vi "Validate IP Address.vi"(4 "Error In":errorcluster, 5 "IP Address":string) -> (0 "Error Out":errorcluster, 1 "IP Address Out":string)   [LabVIEW 2013]
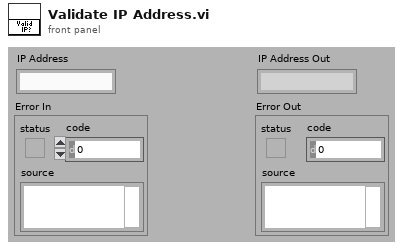
[diagram p1: front panel]
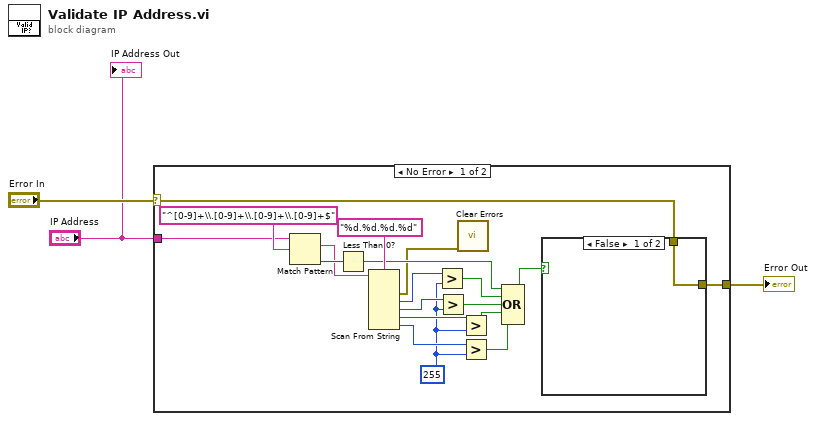
[diagram p0: block diagram]
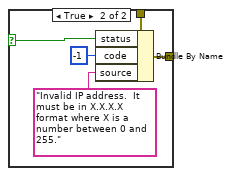
[diagram p2: hidden frame]
diagram:
  n1 = case shown="No Error" "Error In" {
    selector: "Error In" -> [w19 w29]
    tunnel: [w20 w29] -> w3
    tunnel: "IP Address" -> [w18 _]
    frame No Error {
      w12 = 255
      n2 = Match Pattern(string=w18, regular expression="^[0-9]+\\.[0-9]+\\.[0-9]+\\.[0-9]+$") -> (match substring=w7:string, offset past match=w21:i32)  [unwired: 1 in, 2 out]
      n3 = Less Than 0?(x=w21) -> (x < 0?=w6:bool)
      n4 = Scan From String(format string="%d.%d.%d.%d", input string=w7) -> (error out=w4:errorcluster, output 1=w16:i32, output 2=w15:i32, output 3=w14:i32, output 4=w13:i32)  [unwired: 6 in, 2 out]
      n5 = Greater?(x=w16, y=w12) -> (0:w11:bool)
      n6 = Greater?(x=w15, y=w12) -> (0:w10:bool)
      n7 = call <vilib>:"Clear Errors.vi"("error in (no error)"=w4) -> ()  [unwired: 6 in, 1 out]
      n8 = Greater?(x=w14, y=w12) -> (0:w9:bool)
      n9 = Greater?(x=w13, y=w12) -> (0:w8:bool)
      n10 = Compound Arithmetic op=OR(w6, w11, w10, w9, w8) -> (w5:bool)
      n11 = case shown="False" w5 {
        selector: w5 -> [_ w27]
        tunnel: [w23 w28] -> w20
        tunnel: w19 -> [w23 w24]
        frame False {
        }
        frame True {
          n12 = Bundle By Name(cluster=w24, "status"=w27, "code"=-1, "source"="Invalid IP address.  It must be in X.X.X.X format where X is a number between 0 and 255.") -> (w28:errorcluster)
        }
      }
    }
    frame Error {
    }
  }
  "Error Out" <- w3
  "IP Address Out" <- "IP Address"
